vi "FGV.vi"(6 "Write":bool, 10 "Numeric":i32) -> (2 "NumericOut":i32)   [LabVIEW 2014]
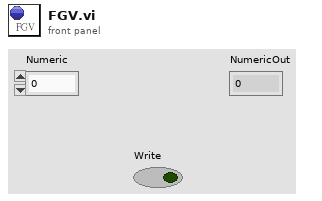
[diagram p1: front panel]
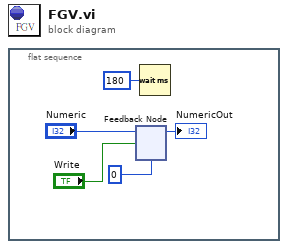
[diagram p0: block diagram]
diagram:
  n1 = flat-sequence {
    frame #0 {
      n2 = feedback #1(0) -> (→"NumericOut":i32)
      n3 = feedback-in #1("Numeric", "Write") -> ()
      n4 = Wait (ms)(milliseconds to wait=u32 180) -> ()  [unwired: 1 out]
    }
  }
